vi "EKGFIlter.vi"(9 "dt":dbl, 10 "Input EKG":dbl[](array[numeric])) -> (2 "EKG Out":dbl[](array[numeric]))   [LabVIEW 2022 SP3]
uses:
  <vilib>/Analysis/1siggen.llb/General Aperiodic Triangle.vi
  <vilib>/Analysis/NI_AALBase.lvlib
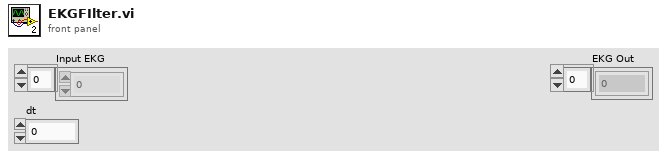
[diagram p1: front panel]
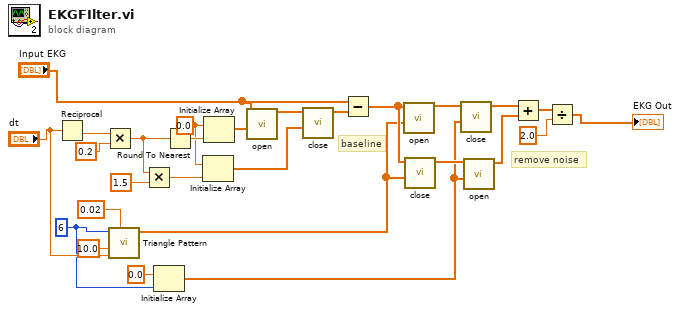
[diagram p0: block diagram]
diagram:
  w1 = 6 ("samples")
  w21 = 0.0 ("element")
  # "remove noise"
  # "baseline"
  n1 = Reciprocal(x="dt") -> (1/x=w27:dbl)
  n2 = Multiply(x=w27, y=0.2) -> (x*y=w24:dbl)
  n3 = call <vilib>:"Triangle Pattern.vi"("width (s)"=0.02, "delta t (s)"="dt", "amplitude"=10.0, "samples"=w1) -> ("Triangle Pattern"=w11:dbl[])  [unwired: 2 in, 5 out]
  n4 = Multiply(x=w24, y=1.5) -> (x*y=w22:dbl)
  n5 = Initialize Array(0.0 ("element"), w1) -> (w9:dbl[])
  n6 = Round To Nearest(number=w24) -> (nearest integer value=w23:dbl)
  n7 = Initialize Array(w21, w22) -> (w18:dbl[])
  n8 = Initialize Array(w21, w23) -> (w20:dbl[])
  n9 = call "open.vi"("structure element"=w20, "x"="Input EKG") -> ("filterd x"=w19:dbl[])  [unwired: 9 out]
  n10 = call "close.vi"("structure element"=w18, "x"=w19) -> ("filterd x"=w17:dbl[])  [unwired: 9 out]
  n11 = Subtract(x="Input EKG", y=w17) -> (x-y=w12:dbl[])
  n12 = call "open.vi"("structure element"=w11, "x"=w12) -> ("filterd x"=w13:dbl[])  [unwired: 9 out]
  n13 = call "close.vi"("structure element"=w11, "x"=w12) -> ("filterd x"=w10:dbl[])  [unwired: 9 out]
  n14 = call "close.vi"("structure element"=w9, "x"=w13) -> ("filterd x"=w8:dbl[])  [unwired: 9 out]
  n15 = call "open.vi"("structure element"=w9, "x"=w10) -> ("filterd x"=w7:dbl[])  [unwired: 9 out]
  n16 = Add(x=w8, y=w7) -> (x+y=w6:dbl[])
  n17 = Divide(x=w6, y=2.0 ("width (s)")) -> (x/y=→"EKG Out":dbl[])
